vi "Main.vi"() -> ()   [LabVIEW 2015]
uses:
  TypDefs/Loop States.ctl
  TypDefs/Loop Data.ctl
panel:
  in  "device name":tag="myDAQ1"
  in  "Exit Button":bool
  in  "Start Button":bool
  out "Status":string
  in  "Clear Button":bool
  in  "Save Button":bool
  out "XY Graph":cluster{"X":dbl[], "Y":dbl[]}(graph)
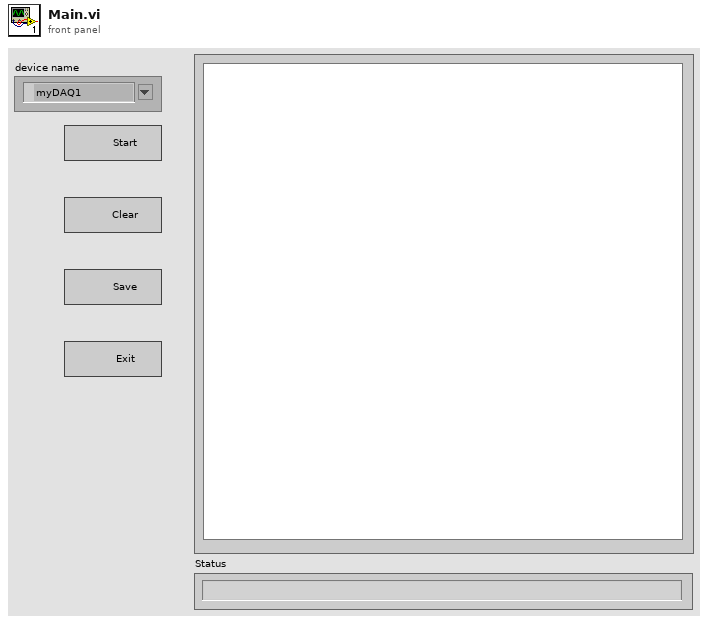
[diagram p1: front panel]
types:
  T1 = typedef "Loop Data.ctl" = cluster{"Status":string, "Graph Data":cluster{"X":dbl[], "Y":dbl[]}, "Recording Status":bool}
  T2 = typedef "Loop States.ctl" = enum16{"Error", "Wait for events", "Measure positions", "Update UI", "Initialization"}
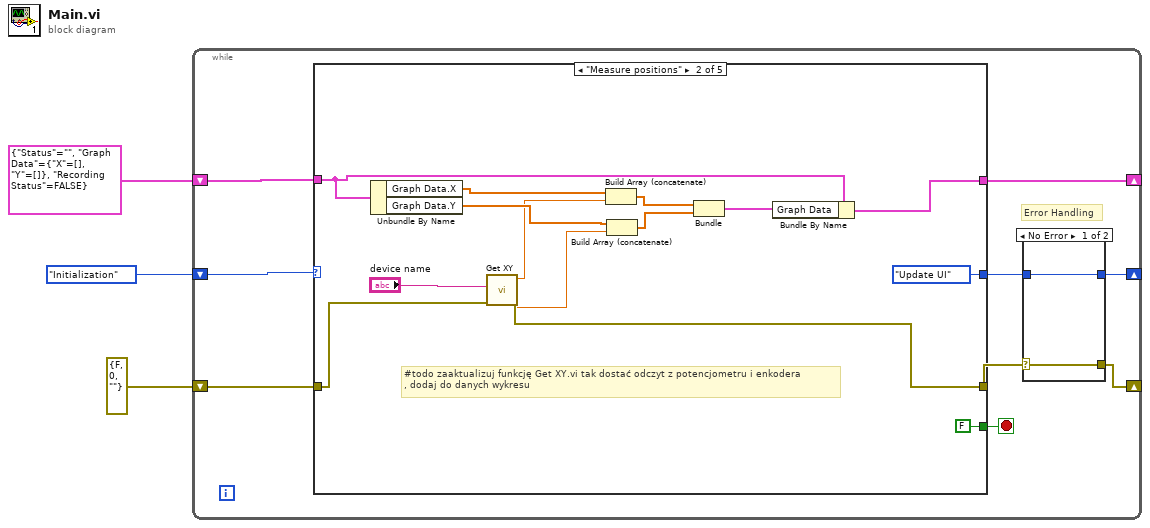
[diagram p0: block diagram]
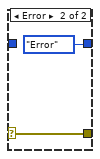
[diagram p2: hidden frame]
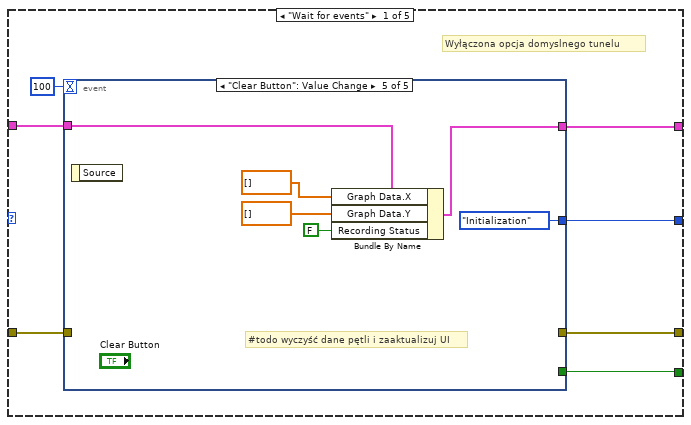
[diagram p3: hidden frame]
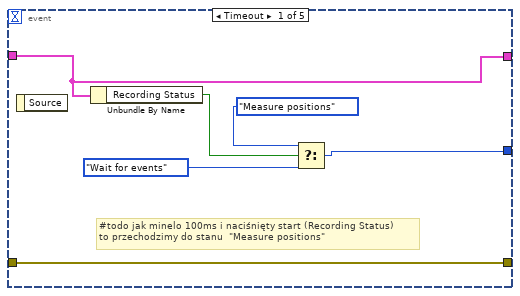
[diagram p4: hidden frame]
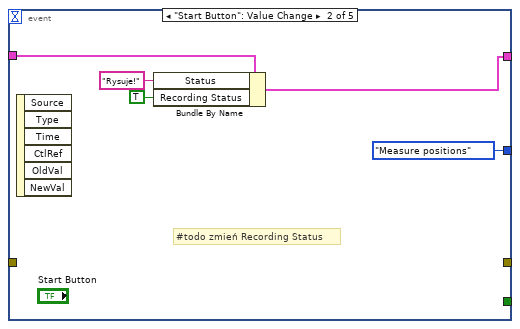
[diagram p5: hidden frame]
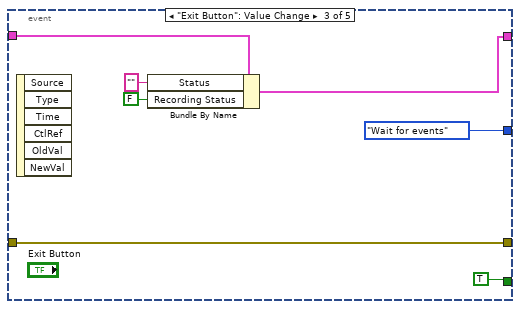
[diagram p6: hidden frame]
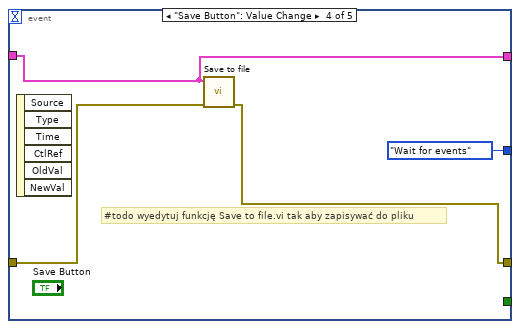
[diagram p7: hidden frame]
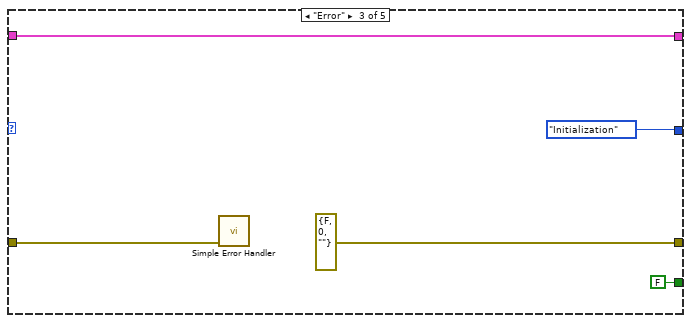
[diagram p8: hidden frame]
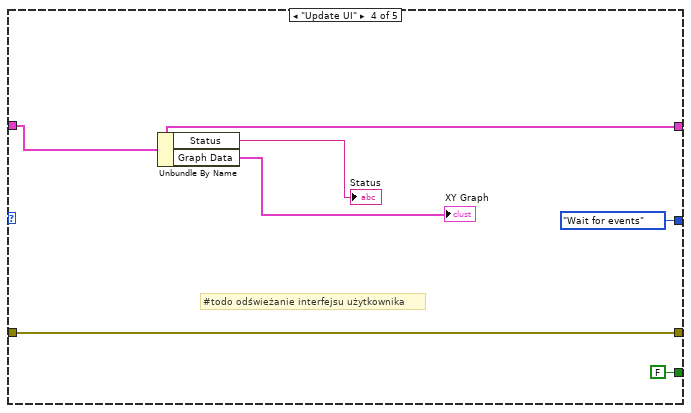
[diagram p9: hidden frame]
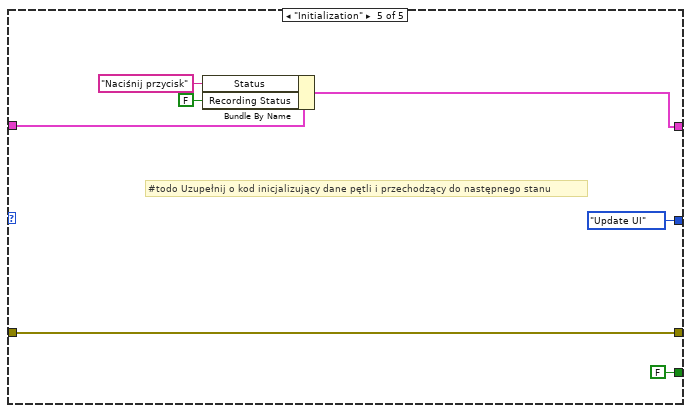
[diagram p10: hidden frame]
diagram:
  n1 = while {
    shift-right: [w10] -> _
    shift-left: T1 {"Status"="", "Graph Data"={"X"=[], "Y"=[]}, "Recording Status"=FALSE} -> [w11]
    shift-right: [w5] -> _
    shift-left: Loop_States."Initialization" -> [w12]
    shift-right: [w4] -> _
    shift-left: errorcluster {"status"=FALSE, "code"=0, "source"=""} ("error constant") -> [w8]
    stop <- w9 stop-if-true
    # "Error Handling"
    n2 = case shown="\"Measure positions\"" w12 {
      tunnel: w11 -> [w22 w62 w67 w74 w82]
      tunnel: [w20 w64 w67 w74 w81] -> w10
      tunnel: [w19 FALSE FALSE FALSE FALSE] -> w9
      tunnel: [w21 Loop_States."Update UI" Loop_States."Initialization" Loop_States."Wait for events" Loop_States."Update UI"] -> w6
      tunnel: w8 -> [w18 w57 w69 w75 w78]
      tunnel: [w17 w56 errorcluster {"status"=FALSE, "code"=0, "source"=""} ("error constant") w75 w78] -> w7
      frame "Wait for events" {
        # "Wyłączona opcja domyslnego tunelu"
        n3 = event shown="[4] \"Clear Button\": Value Change" {
          selector: _ -> [_ _ _ _ _]
          dyn-events: _ -> [_ _ _ _ _]
          timeout: 100 -> [_ _ _ _ _]
          tunnel: w22 -> [w24 w33 w38 w42 w51]
          tunnel: [w25 Loop_States."Measure positions" Loop_States."Wait for events" Loop_States."Wait for events" Loop_States."Initialization"] -> w21
          tunnel: [w24 w32 w37 w42 w50] -> w20
          tunnel: [_ _ TRUE _ _] -> w19
          tunnel: w18 -> [w29 _ w39 w44 _]
          tunnel: [w29 _ w39 w43 _] -> w17
          event Timeout {
            # "#todo jak minelo 100ms i naciśnięty start (Recording Status) \nto przechodzimy do stanu  \"Measure positions\""
            n4 = event-data() -> ()  [unwired: 1 in, 1 out]
            n5 = Unbundle By Name(w24) -> ("Recording Status"=w28:bool)
            n6 = Select(t=Loop_States."Measure positions", s=w28, f=Loop_States."Wait for events") -> (s? t:f=w25:T2)
          }
          event "Start Button": Value Change {
            # "#todo zmień Recording Status"
            n7 = event-data() -> ()  [unwired: 1 in, 6 out]
            n8 = Bundle By Name(cluster=w33, "Status"="Rysuje!", "Recording Status"=TRUE) -> (w32:T1)
          }
          event "Exit Button": Value Change {
            n9 = event-data() -> ()  [unwired: 1 in, 6 out]
            n10 = Bundle By Name(cluster=w38, "Status"="", "Recording Status"=FALSE) -> (w37:T1)
          }
          event "Save Button": Value Change {
            # "#todo wyedytuj funkcję Save to file.vi tak aby zapisywać do pliku"
            n11 = event-data() -> ()  [unwired: 1 in, 6 out]
            n12 = call "Save to file.vi"("error in (no error)"=w44, "Loop Data"=w42) -> ("error out"=w43:errorcluster)  [unwired: 9 in]
          }
          event "Clear Button": Value Change {
            # "#todo wyczyść dane pętli i zaaktualizuj UI"
            n13 = event-data() -> ()  [unwired: 1 in, 1 out]
            n14 = Bundle By Name(cluster=w51, "Graph Data.X"=dbl[] [], "Graph Data.Y"=dbl[] [], "Recording Status"=FALSE) -> (w50:T1)
          }
        }
      }
      frame "Measure positions" {
        # "#todo zaaktualizuj funkcję Get XY.vi tak dostać odczyt z potencjometru i enkodera \n, dodaj do danych wykresu"
        n15 = Unbundle By Name(w62) -> ("Graph Data.X"=w61:dbl[], "Graph Data.Y"=w60:dbl[])
        n16 = call "Get XY.vi"("error in"=w57, "device name"="device name") -> ("error out"=w56:errorcluster, "Y"=w54:dbl, "X"=w53:dbl)  [unwired: 7 in]
        n17 = Build Array (concatenate)(w61, w53) -> (w59:dbl[])
        n18 = Build Array (concatenate)(w60, w54) -> (w58:dbl[])
        n19 = Bundle(w59, w58) -> (w52:cluster{dbl[], dbl[]})  [unwired: 1 in]
        n20 = Bundle By Name(cluster=w62, "Graph Data"=w52) -> (w64:T1)
      }
      frame "Error" {
        n21 = call <vilib>:"Simple Error Handler.vi"("error in (no error)"=w69) -> ()  [unwired: 4 in, 5 out]
      }
      frame "Update UI" {
        # "#todo odświeżanie interfejsu użytkownika"
        n22 = Unbundle By Name(w74) -> ("Status"=→"Status":string, "Graph Data"=→"XY Graph":cluster{"X":dbl[], "Y":dbl[]})
      }
      frame "Initialization" {
        # "#todo Uzupełnij o kod inicjalizujący dane pętli i przechodzący do następnego stanu"
        n23 = Bundle By Name(cluster=w82, "Status"="Naciśnij przycisk", "Recording Status"=FALSE) -> (w81:T1)
      }
    }
    n24 = case shown="No Error" w7 {
      selector: w7 -> [w13 w15]
      tunnel: w6 -> [w14 _]
      tunnel: [w14 Loop_States."Error"] -> w5
      tunnel: [w13 w15] -> w4
      frame No Error {
      }
      frame Error {
      }
    }
  }
